vi "4_5.vi"() -> ()   [LabVIEW 2015]
panel:
  in  "stop":bool
  out "operator":string
  out "Result":dbl
  in  "B":dbl
  in  "A":dbl
  in  "Enum":T1(ring)
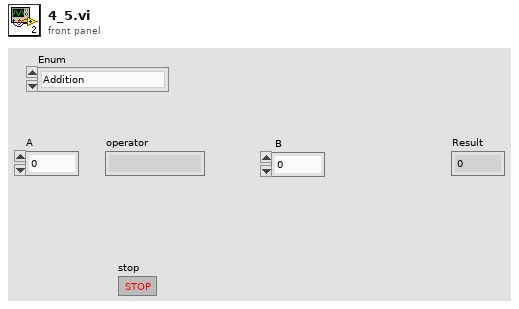
[diagram p1: front panel]
types:
  T1 = enum16{"Addition", "Subtract", "Division", "Multiply"}
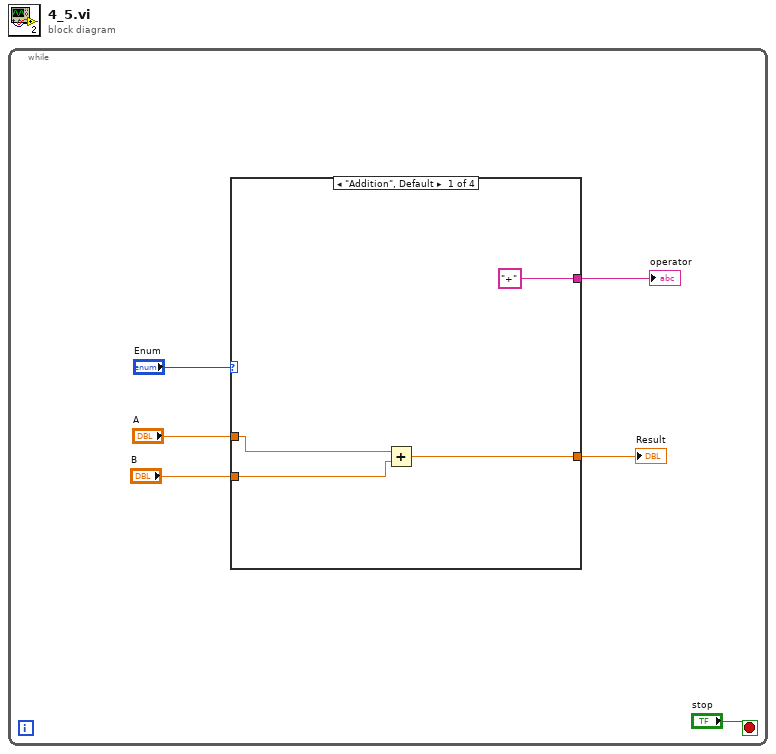
[diagram p0: block diagram]
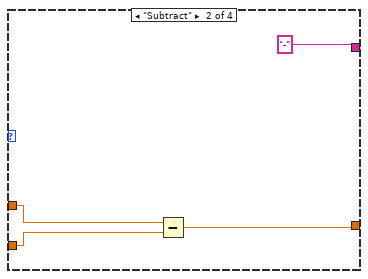
[diagram p2: hidden frame]
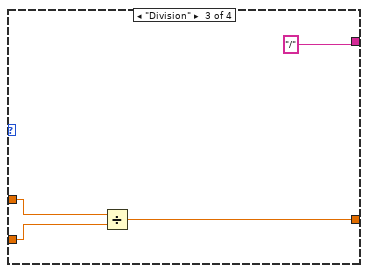
[diagram p3: hidden frame]
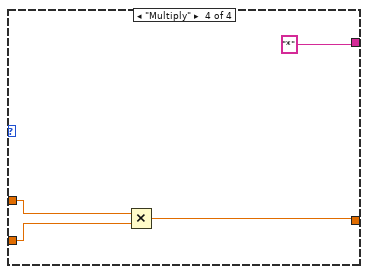
[diagram p4: hidden frame]
diagram:
  n1 = while {
    stop <- "stop" stop-if-true
    n2 = case shown="\"Addition\", Default" "Enum" {
      tunnel: "A" -> [w10 w14 w18 w22]
      tunnel: "B" -> [w9 w13 w17 w21]
      tunnel: ["+" "-" "/" "*"] -> w3
      tunnel: [w7 w12 w16 w20] -> w2
      frame "Addition", Default {
        n3 = Add(x=w10, y=w9) -> (x+y=w7:dbl)
      }
      frame "Subtract" {
        n4 = Subtract(x=w14, y=w13) -> (x-y=w12:dbl)
      }
      frame "Division" {
        n5 = Divide(x=w18, y=w17) -> (x/y=w16:dbl)
      }
      frame "Multiply" {
        n6 = Multiply(x=w22, y=w21) -> (x*y=w20:dbl)
      }
    }
    "Result" <- w2
    "operator" <- w3
  }
